vi "Calibration_Main.vi"() -> ()   [LabVIEW 2017]
uses:
  <vilib>/userdefined/High Color/IMAQdx.ctl
  <vilib>/vision/Calibration.llb/Error Statistics.ctl
  Integration/Kicker-XY loop integration/Flow Control Enum.ctl
  <vilib>/vision/NI_Vision_Development_Module.lvlib
panel:
  in  "Tab Control":T1(tab)
  in  "Rebound Only":bool
  out "Kick Success":bool
  out "TrajectorySuccess":bool
  in  "Kick":bool
  in  "stop":bool
  out "error out":errorcluster
  out "ImageOut":T2(plugin-control)
  in  "Session In":T3
  out "X Speed PID":cluster{"Speed SP":dbl, "Speed PV":dbl}(graph)
  out "Y Speed PID":cluster{"Speed SP":dbl, "Speed PV":dbl}(graph)
  out "State":T4(ring)
  out "Kicked":bool
  out "Image":T2(plugin-control)
  out "Datum Check":T5
  in  "EnergyFudgeFactor":dbl
  out "Horizontal Edges":T6(array[cluster]) {"Point2 (Real-World)"."Y" format="%.2f"; "Point2 (Real-World)"."X" format="%.2f"; "Point1 (Real-World)"."Y" format="%.2f"; "Point1 (Real-World)"."X" format="%.2f"; "Point2 (Pixels)"."Y" format="%.2f"; "Point2 (Pixels)"."X" format="%.2f"; "Point1 (Pixels)"."Y" format="%.2f"; "Point1 (Pixels)"."X" format="%.2f"}
  out "Vertical Edges":T6(array[cluster]) {"Point2 (Real-World)"."Y" format="%.2f"; "Point2 (Real-World)"."X" format="%.2f"; "Point1 (Real-World)"."Y" format="%.2f"; "Point1 (Real-World)"."X" format="%.2f"; "Point2 (Pixels)"."Y" format="%.2f"; "Point2 (Pixels)"."X" format="%.2f"; "Point1 (Pixels)"."Y" format="%.2f"; "Point1 (Pixels)"."X" format="%.2f"}
  out "Players":T7(array[cluster]) {"Position"."Y" format="%.2f"; "Position"."X" format="%.2f"}
  out "ChosenAngle":dbl
  out "ChosenPathIdx":i32
  out "ChosenEnergy":dbl
  out "Kicker XY":cluster{dbl, dbl}
  out "Puck":T7(array[cluster]) {"Position"."Y" format="%.2f"; "Position"."X" format="%.2f"}
  out "Image Out":T2(plugin-control)
  out "X 2":sgl
  out "Y 2":sgl
  out "error out 2":errorcluster
  out "Y distance Out":dbl
  out "All Edges Found":bool
  out "X distance":dbl
  out "Histogram Graph":cluster{dbl[], dbl[]}(graph)
  in  "Brightness Input":i64(slide) scale=0.0..255.0
  in  "Contrast Input":dbl(slide) scale=0.0..1.0
  in  "Threshold Input":sgl(slide) scale=0.0..255.0
  in  "Stop":bool
  out "Camera Setup Error":errorcluster
  out "Threshold Image":T2(plugin-control)
  out "Before Image":T2(plugin-control)
  out "Histogram Statistics":T8
  out "Quality Check Variables":T9
  in  "Reference":bool
  in  "stop 2":bool
  out "Image 2":T2(plugin-control)
  in  "Calibrate":bool
  in  "Grid Descriptor":cluster{"X Step":sgl, "Y Step":sgl, "Unit":T10}={"X Step"=5.0, "Y Step"=5.0, "Unit"=enum."Millimeter"}
  in  "File Path":path
  out "Calibration Error":errorcluster
  out "Corrected Image":T2(plugin-control)
  out "Y":sgl
  out "X":sgl
  out "Error Statistics":T11
  # "0.6"
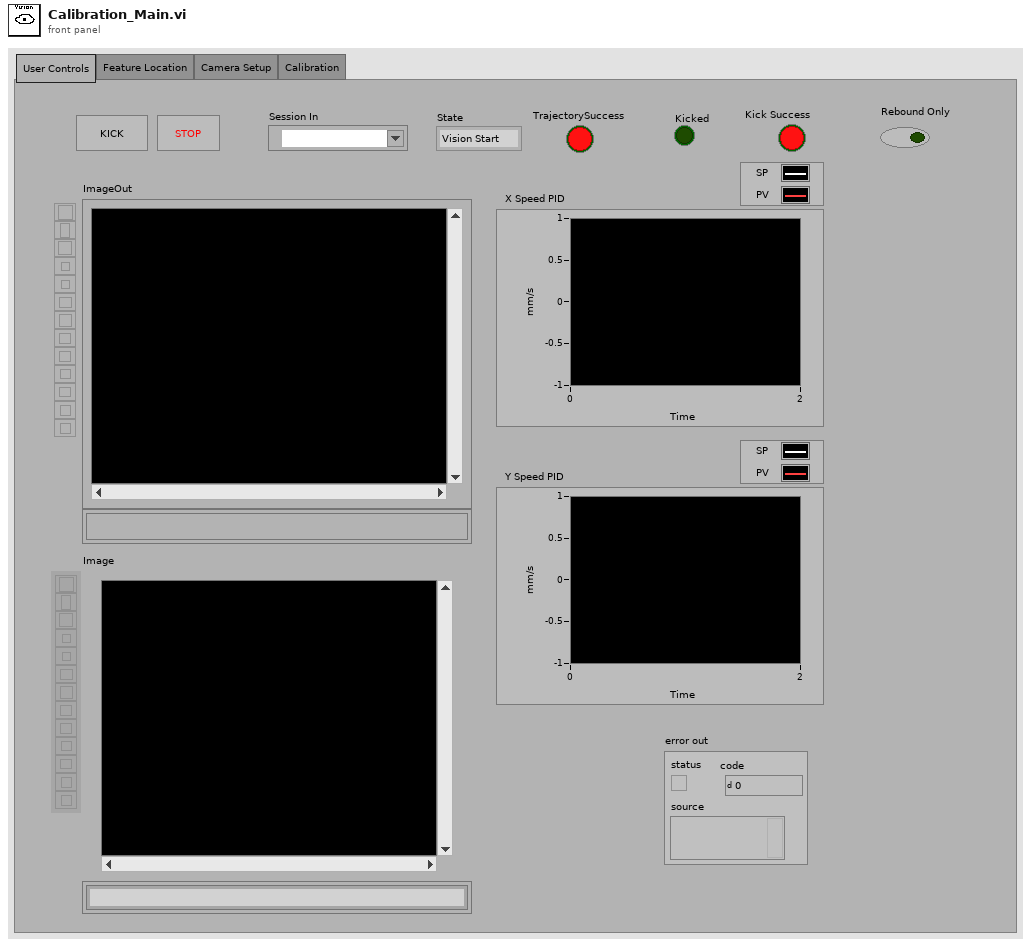
[diagram p1: front panel]
types:
  T1 = enum32{"User Controls", "Feature Location", "Camera Setup", "Calibration"}
  T2 = typedef "IMAQ Image.ctl" = refnum<image>
  T3 = typedef "IMAQdx.ctl" = refnum<k21>
  T4 = enum16{"Vision Start", "Vision End", "Plotting", "Wait"}
  T5 = cluster{"X Coord Correct":bool, "Y Coord Correct":bool}
  T6 = cluster{"Point1 (Pixels)":cluster{"X":sgl, "Y":sgl}, "Point2 (Pixels)":cluster{"X":sgl, "Y":sgl}, "Point1 (Real-World)":cluster{"X":sgl, "Y":sgl}, "Point2 (Real-World)":cluster{"X":sgl, "Y":sgl}, "Angle (Pixel)":dbl, "Angle (Real-World)":dbl, "Score":dbl, "Straightness":dbl, "Average SNR (db)":dbl, "Calibration Valid":bool}[]
  T7 = cluster{"Position":cluster{"X":sgl, "Y":sgl}, "Radius":dbl, "Score":dbl}[]
  T8 = cluster{"Mean Value":sgl, "Standard  Variation":sgl, "Range":sgl}
  T9 = cluster{"Mean +":dbl, "Mean -":dbl, "Within Range":bool}
  T10 = typedef "Image Unit" = enum32{"Undefined", "Angström", "Micrometer", "Millimeter", "Centimeter", "Meter", "Kilometer", "Microinch", "Inch", "Feet", "Nautical miles", "Standard miles", "Steps"}
  T11 = typedef "Error Statistics.ctl" = cluster{"Mean Error":dbl, "Maximum Error":dbl, "Standard Deviation":dbl, "% Distortion":dbl}
  T12 = cluster{"Brightness":i64, "Contrast":dbl, "Threshold":sgl}
  T13 = cluster{"XCoordCorrect":bool, "YCoordCorrect":bool}
  T14 = typedef "IMAQ Coordinate System" = cluster{"Reference System":cluster{"Origin":cluster{"X":sgl, "Y":sgl}, "Angle (deg)":sgl, "Axis Reference":u32}, "Measurement System":cluster{"Origin":cluster{"X":sgl, "Y":sgl}, "Angle (deg)":sgl, "Axis Reference":u32}}
  T15 = cluster{"Circles[0]":cluster{"Position":cluster{"X":sgl, "Y":sgl}, "Radius":dbl, "Score":dbl}, "Circles[1]":cluster{"Position":cluster{"X":sgl, "Y":sgl}, "Radius":dbl, "Score":dbl}, "Circles[2]":cluster{"Position":cluster{"X":sgl, "Y":sgl}, "Radius":dbl, "Score":dbl}, "Circles[3]":cluster{"Position":cluster{"X":sgl, "Y":sgl}, "Radius":dbl, "Score":dbl}, "Circles[4]":cluster{"Position":cluster{"X":sgl, "Y":sgl}, "Radius":dbl, "Score":dbl}, "Circles[5]":cluster{"Position":cluster{"X":sgl, "Y":sgl}, "Radius":dbl, "Score":dbl}, "Circles[6]":cluster{"Position":cluster{"X":sgl, "Y":sgl}, "Radius":dbl, "Score":dbl}, "Circles[7]":cluster{"Position":cluster{"X":sgl, "Y":sgl}, "Radius":dbl, "Score":dbl}, "Circles[8]":cluster{"Position":cluster{"X":sgl, "Y":sgl}, "Radius":dbl, "Score":dbl}}
  T16 = cluster{"X Coord":dbl, "Y Coord":dbl, "Energy":dbl, "Theta Angle":dbl}
  T17 = cluster{"Ptwx":dbl[], "Ptwy":dbl[], "Ptfx":dbl[], "Ptfy":dbl[], "DorR":i32[]}
  T18 = cluster{"X Axis":cluster{"Displacement":dbl, "Speed SP":dbl, "Speed PV":dbl, "Acceleration":dbl}, "Y Axis":cluster{"Displacement":dbl, "Speed SP":dbl, "Speed PV":dbl, "Acceleration":dbl}, "XY Complete?":bool}
  T19 = cluster{"Displacement":dbl, "Speed SP":dbl, "Speed PV":dbl, "Acceleration":dbl}
  T20 = typedef "Flow Control Enum.ctl" = enum16{"Update I/O", "Kicker", "XY Drive", "Theta Axis", "Solenoid", "Go Home"}
  T21 = cluster{"Kicked?":bool, "Stop?":bool, "State":T20, "At Home":bool}
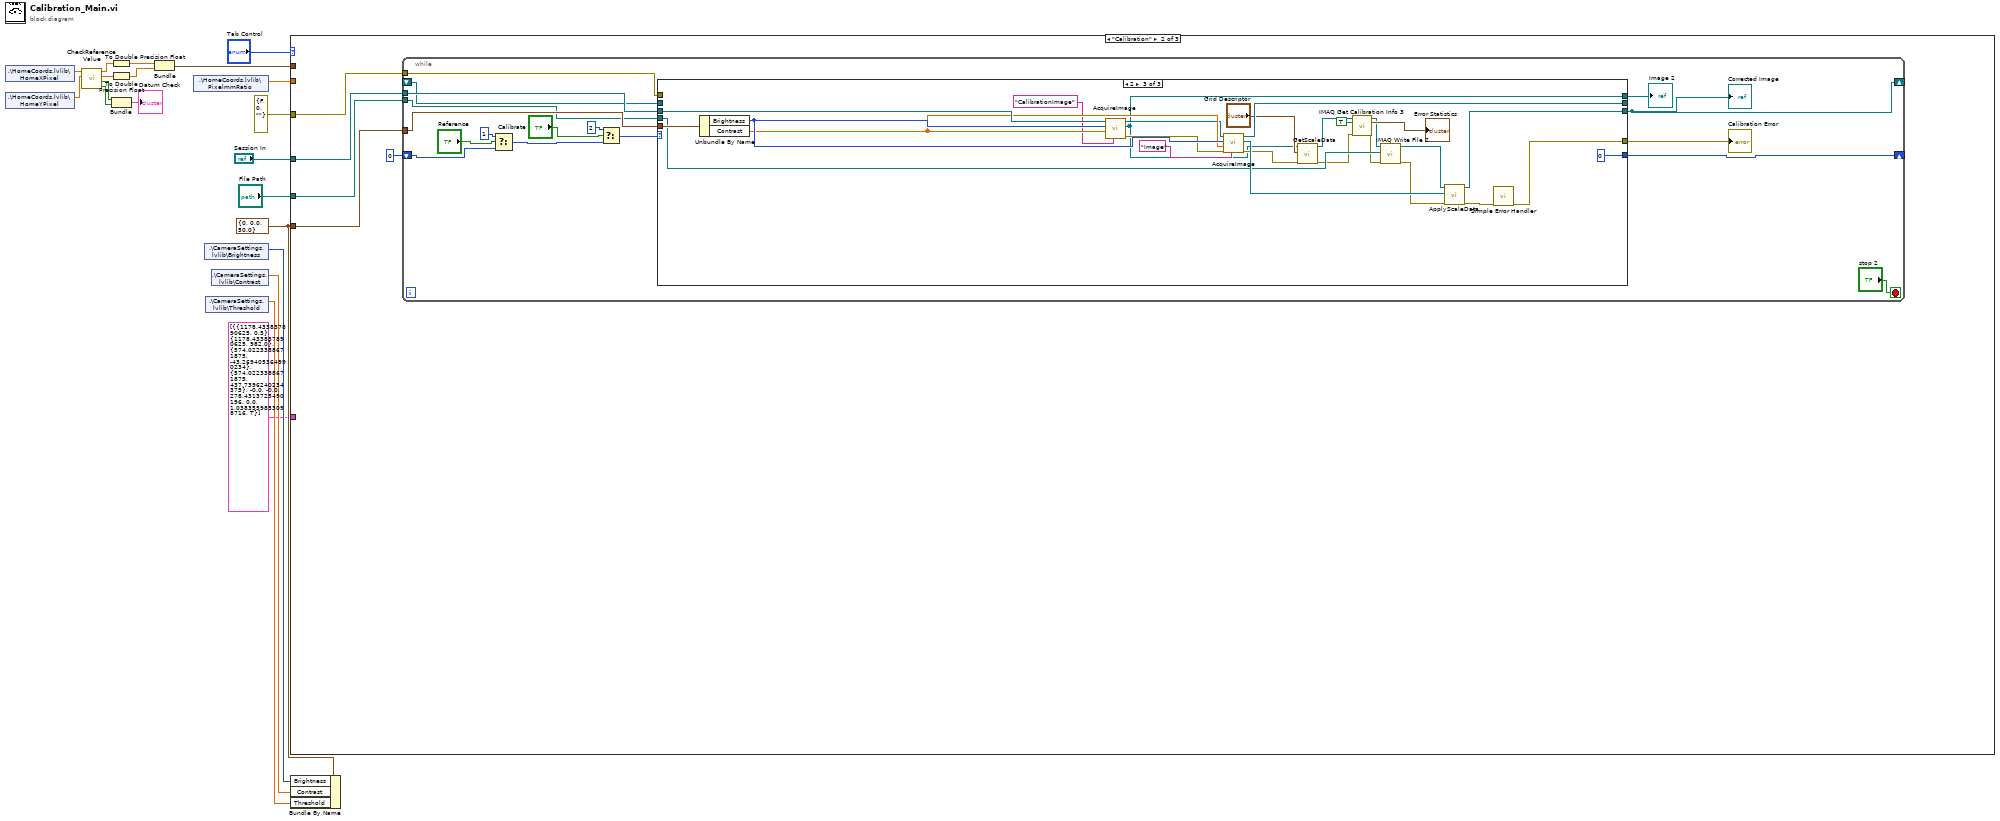
[diagram p0: block diagram]
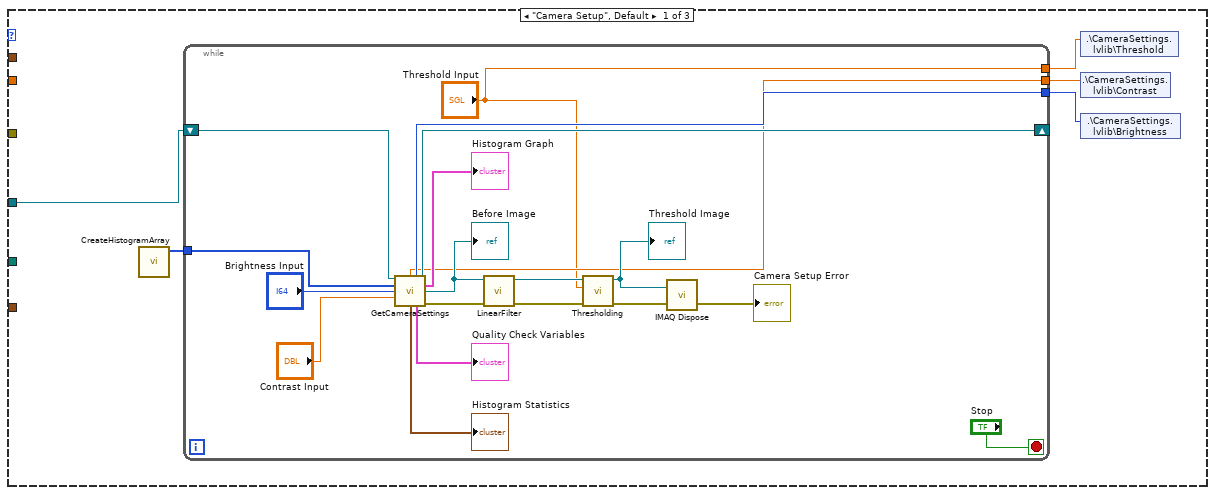
[diagram p2: hidden frame]
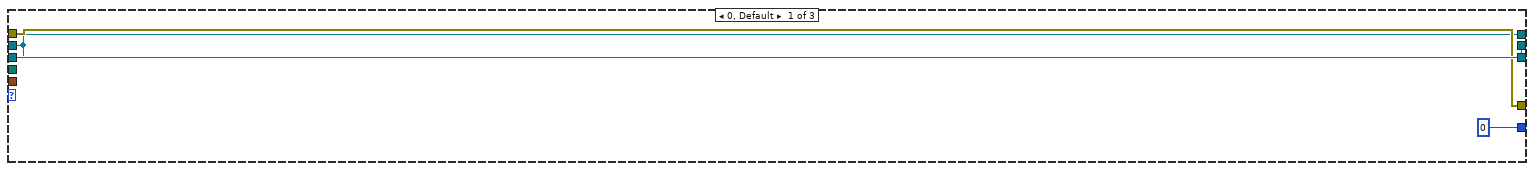
[diagram p3: hidden frame]
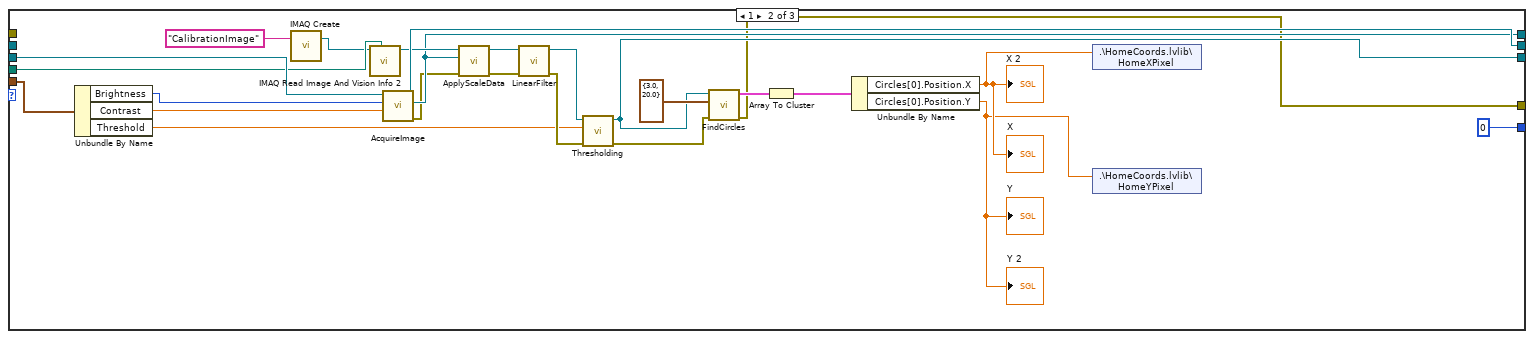
[diagram p4: hidden frame]
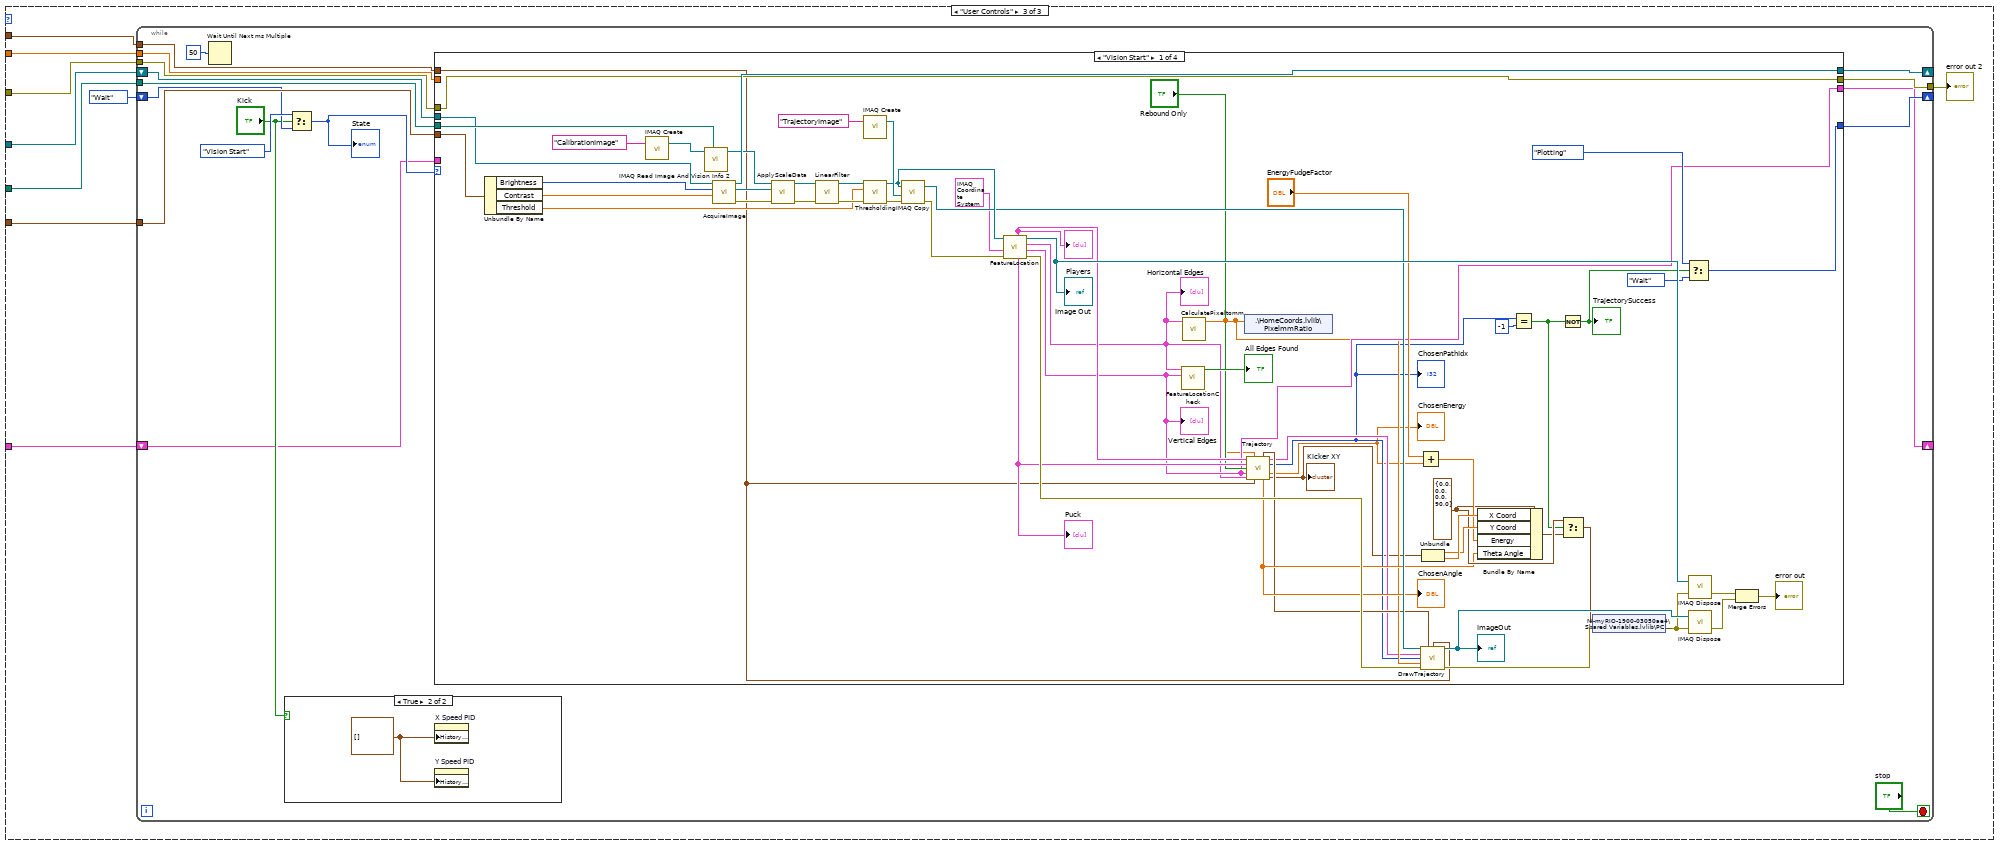
[diagram p5: hidden frame]
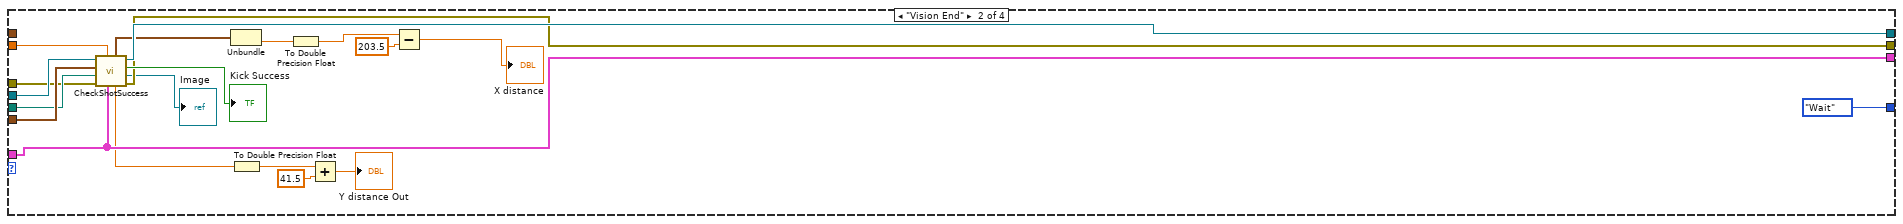
[diagram p7: hidden frame]
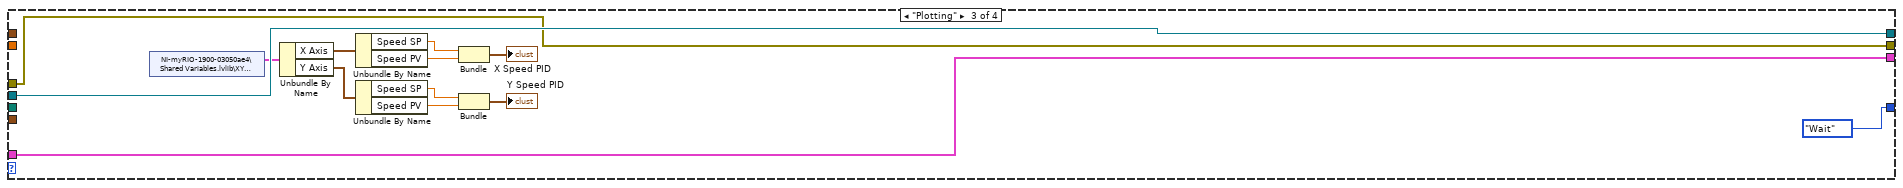
[diagram p8: hidden frame]
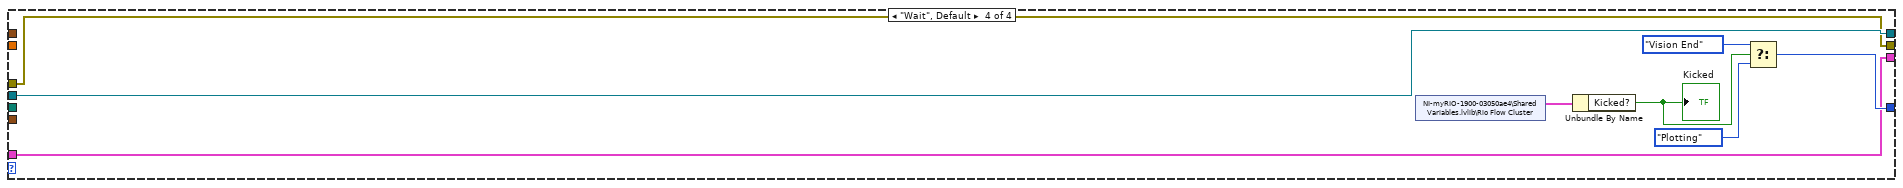
[diagram p9: hidden frame]
diagram:
  w15 = T12 {"Brightness"=0, "Contrast"=0.0, "Threshold"=50.0} ("CameraSettings")
  n1 = shared-variable ".\\HomeCoords.lvlib\\HomeXPixel"() -> (w10:sgl)  [unwired: 1 in, 1 out]
  n2 = shared-variable ".\\HomeCoords.lvlib\\HomeYPixel"() -> (w8:sgl)  [unwired: 1 in, 1 out]
  n3 = call "CheckReferenceValue.vi"("YCoordIn"=w8, "XCoordIn"=w10) -> ("YCoordCorrect"=w2:bool, "XCoordCorrect"=w3:bool, "YCoordOut"=w7:sgl, "XCoordOut"=w9:sgl)  [unwired: 6 in]
  n4 = To Double Precision Float(number=w9) -> (double precision float=w12:dbl)
  n5 = To Double Precision Float(number=w7) -> (double precision float=w11:dbl)
  n6 = Bundle("XCoordCorrect"=w3, "YCoordCorrect"=w2) -> (→"Datum Check":T13)  [unwired: 1 in]
  n7 = Bundle(w12, w11) -> (w17:cluster{dbl, dbl})  [unwired: 1 in]
  n8 = shared-variable ".\\HomeCoords.lvlib\\PixelmmRatio"() -> (w5:dbl)  [unwired: 1 in, 1 out]
  n9 = shared-variable ".\\CameraSettings.lvlib\\Brightness"() -> (w16:i64)  [unwired: 1 in, 1 out]
  n10 = shared-variable ".\\CameraSettings.lvlib\\Threshold"() -> (w13:sgl)  [unwired: 1 in, 1 out]
  n11 = shared-variable ".\\CameraSettings.lvlib\\Contrast"() -> (w14:dbl)  [unwired: 1 in, 1 out]
  n12 = case shown="\"Calibration\"" "Tab Control" {
    tunnel: "Session In" -> [w24 w49 w130]
    tunnel: w15 -> [_ w48 w128]
    tunnel: "File Path" -> [_ w47 w129]
    tunnel: errorcluster {"status"=FALSE, "code"=0, "source"=""} ("error out") -> [_ w45 w126]
    tunnel: w17 -> [_ _ w127]
    tunnel: w5 -> [_ _ w123]
    tunnel: T6 [{"Point1 (Pixels)"={"X"=1178.4338, "Y"=0.5}, "Point2 (Pixels)"={"X"=1178.4338, "Y"=982.0}, "Point1 (Real-World)"={"X"=574.02234, "Y"=-43.269405}, "Point2 (Real-World)"={"X"=574.02234, "Y"=437.73962}, "Angle (Pixel)"=-0.0, "Angle (Real-World)"=-0.0, "Score"=278.4313725490196, "Straightness"=0.0, "Average SNR (db)"=1.0383559853098716, "Calibration Valid"=TRUE}] ("Vertical Edges 2") -> [_ _ w122]
    frame "Camera Setup", Default {
      n13 = call "CreateHistogramArray.vi"() -> ("Array"=w25:i32[])  [unwired: 11 in]
      n14 = while {
        shift-right: [w34] -> _
        shift-left: w24 -> [w42]
        tunnel: w25 -> [w41]
        tunnel: [w29] -> w22
        tunnel: ["Threshold Input"] -> w21
        tunnel: [w30] -> w23
        stop <- "Stop" stop-if-true
        n15 = call "GetCameraSettings.vi"("Session In"=w42, "Array"=w41, "Brightness"="Brightness Input", "Contrast"="Contrast Input") -> ("Contrast"=w29:dbl, "Brightness"=w30:i64, "Session Out"=w34:T3, "Histogram Graph"=→"Histogram Graph":cluster{dbl[], dbl[]}, "Image"=w33:T2, "Histogram Statistics"=→"Histogram Statistics":T8, "Quality Check Variables"=→"Quality Check Variables":T9, "error out"=w32:errorcluster)  [unwired: 4 in]
        "Before Image" <- w33
        n16 = call "LinearFilter.vi"("error in (no error)"=w32, "Image Src"=w33) -> ("error out"=w37:errorcluster, "Image"=w38:T2)  [unwired: 8 in]
        n17 = call "Thresholding.vi"("error in (no error)"=w37, "Threshold Value"="Threshold Input", "Image Src"=w38) -> ("error out"=w36:errorcluster, "Image"=w35:T2)  [unwired: 7 in]
        "Threshold Image" <- w35
        n18 = call "IMAQ Dispose"("Image"=w35, "error in (no error)"=w36) -> ("error out"=→"Camera Setup Error":errorcluster)  [unwired: 4 in]
      }
      n19 = shared-variable ".\\CameraSettings.lvlib\\Threshold"(w21) -> ()  [unwired: 1 in, 1 out]
      n20 = shared-variable ".\\CameraSettings.lvlib\\Contrast"(w22) -> ()  [unwired: 1 in, 1 out]
      n21 = shared-variable ".\\CameraSettings.lvlib\\Brightness"(w23) -> ()  [unwired: 1 in, 1 out]
    }
    frame "Calibration" {
      n22 = while {
        tunnel: w49 -> [w66]
        tunnel: w48 -> [w65]
        tunnel: w47 -> [w63]
        shift-right: [w62] -> _
        shift-left: 0 -> [w56]
        shift-right: [w50] -> _
        shift-left: _ -> [w53]
        tunnel: w45 -> [w54]
        stop <- "stop 2" stop-if-true
        n23 = Select(t=1, s="Reference", f=w56) -> (s? t:f=w59:i32)
        n24 = Select(t=2, s="Calibrate", f=w59) -> (s? t:f=w55:i32)
        n25 = case shown="2" w55 {
          tunnel: w66 -> [w70 w93 w121]
          tunnel: w65 -> [_ w91 w120]
          tunnel: [w70 w92 w113] -> _
          tunnel: w63 -> [_ w89 w105]
          tunnel: [w68 w73 w115] -> w52
          tunnel: [w67 w74 w106] -> w50
          tunnel: [0 0 0] -> w62
          tunnel: w54 -> [w68 _ _]
          tunnel: w53 -> [w67 _ _]
          tunnel: [w67 w85 w104] -> w51
          frame 0, Default {
          }
          frame 1 {
            n26 = Unbundle By Name(w91) -> ("Brightness"=w95:i64, "Contrast"=w94:dbl, "Threshold"=w79:sgl)
            n27 = call "IMAQ Create"("Image Name"="CalibrationImage") -> ("New Image"=w87:T2)  [unwired: 4 in, 1 out]
            n28 = call "IMAQ Read Image And Vision Info 2"("File Path"=w89, "Image"=w87) -> ("Image Out"=w86:T2)  [unwired: 7 in, 2 out]
            n29 = call "AcquireImage.vi"("Contrast"=w94, "Brightness"=w95, "Session In"=w93) -> ("error out"=w82:errorcluster, "Image"=w85:T2, "Session Out"=w92:T3)  [unwired: 5 in]
            n30 = call "ApplyScaleData.vi"("error in (no error)"=w82, "ImageIn"=w85, "CalibImage"=w86) -> ("error out"=w81:errorcluster, "Corrected Image"=w84:T2)  [unwired: 7 in]
            n31 = call "LinearFilter.vi"("error in (no error)"=w81, "Image Src"=w84) -> ("error out"=w80:errorcluster, "Image"=w83:T2)  [unwired: 8 in]
            n32 = call "Thresholding.vi"("error in (no error)"=w80, "Threshold Value"=w79, "Image Src"=w83) -> ("error out"=w77:errorcluster, "Image"=w74:T2)  [unwired: 7 in]
            n33 = call "FindCircles.vi"("error in (no error)"=w77, "Circle Descriptor"=cluster{"Min Radius":dbl, "Max Radius":dbl} {"Min Radius"=3.0, "Max Radius"=20.0}, "Image"=w74) -> ("error out"=w73:errorcluster, "Circles"=w76:T7)  [unwired: 6 in, 1 out]
            n34 = Array To Cluster(array=w76) -> (cluster=w75:T15)
            n35 = Unbundle By Name(w75) -> ("Circles[0].Position.X"=w72:sgl, "Circles[0].Position.Y"=w71:sgl)
            "X 2" <- w72
            "Y 2" <- w71
            "Y" <- w71
            "X" <- w72
            n36 = shared-variable ".\\HomeCoords.lvlib\\HomeXPixel"(w72) -> ()  [unwired: 1 in, 1 out]
            n37 = shared-variable ".\\HomeCoords.lvlib\\HomeYPixel"(w71) -> ()  [unwired: 1 in, 1 out]
          }
          frame 2 {
            n38 = Unbundle By Name(w120) -> ("Brightness"=w118:i64, "Contrast"=w117:dbl)
            n39 = call "AcquireImage.vi"("Image Name"="CalibrationImage", "Contrast"=w117, "Brightness"=w118, "Session In"=w121) -> ("error out"=w116:errorcluster, "Image"=w104:T2, "Session Out"=w114:T3)  [unwired: 4 in]
            n40 = call "AcquireImage.vi"("Image Name"="Image", "error in"=w116, "Contrast"=w117, "Brightness"=w118, "Session In"=w114) -> ("error out"=w108:errorcluster, "Image"=w109:T2, "Session Out"=w113:T3)  [unwired: 3 in]
            n41 = call "GetScaleData.vi"("error in (no error)"=w108, "Grid Descriptor"="Grid Descriptor", "Image Src"=w104) -> ("error out"=w99:errorcluster, "Image"=w102:T2)  [unwired: 7 in]
            n42 = call "IMAQ Get Calibration Info 3"("Calibration Template Image"=w102, "Return Error Information (False)"=TRUE, "error in (no error)"=w99) -> ("Calibration Template Image (duplicate)"=w100:T2, "Error Statistics"=→"Error Statistics":T11, "error out"=w98:errorcluster)  [unwired: 4 in, 6 out]
            n43 = call-poly "IMAQ Write File 2"("error in (no error)"=w98, "File Path"=w105, "Image"=w100) -> ("error out"=w97:errorcluster, "Image Out (duplicate)"=w101:T2)  [unwired: 7 in]
            n44 = call "ApplyScaleData.vi"("error in (no error)"=w97, "ImageIn"=w109, "CalibImage"=w101) -> ("error out"=w107:errorcluster, "Corrected Image"=w106:T2)  [unwired: 7 in]
            n45 = call <vilib>:"Simple Error Handler.vi"("error in (no error)"=w107) -> ("error out"=w115:errorcluster)  [unwired: 4 in, 4 out]
          }
        }
        "Calibration Error" <- w52
        "Image 2" <- w51
        "Corrected Image" <- w50
      }
    }
    frame "User Controls" {
      n46 = while {
        shift-right: [w146] -> _
        shift-left: w130 -> [w147]
        tunnel: w129 -> [w144]
        tunnel: w128 -> [w143]
        tunnel: w127 -> [w142]
        shift-right: [w139] -> _
        shift-left: T4."Wait" -> [w138]
        tunnel: w126 -> [w135]
        tunnel: [w134] -> w125
        tunnel: w123 -> [w133]
        shift-right: [w131] -> _
        shift-left: w122 -> [w132]
        stop <- "stop" stop-if-true
        n47 = Wait Until Next ms Multiple(millisecond multiple=u32 50) -> ()  [unwired: 1 out]
        n48 = case shown="True" "Kick" {
          frame False {
          }
          frame True {
            w148 = cluster{"Speed SP":dbl, "Speed PV":dbl}[] [] ("History Data")
            n49 = property on="X Speed PID" class="WFChart (strict)"("History Data"=w148) -> ()  [unwired: 2 in, 2 out]
            n50 = property on="Y Speed PID" class="WFChart (strict)"("History Data"=w148) -> ()  [unwired: 2 in, 2 out]
          }
        }
        n51 = Select(t=T4."Vision Start", s="Kick", f=w138) -> (s? t:f=w140:T4)
        "State" <- w140
        n52 = case shown="\"Vision Start\"" w140 {
          tunnel: w147 -> [w195 w226 w240 w248]
          tunnel: [w204 w225 w240 w248] -> w146
          tunnel: w144 -> [w207 w221 _ _]
          tunnel: w143 -> [w202 w222 _ _]
          tunnel: w142 -> [w156 _ _ _]
          tunnel: [w164 T4."Wait" T4."Wait" w244] -> w139
          tunnel: w135 -> [w163 w220 w230 w247]
          tunnel: [w163 w219 w230 w247] -> w134
          tunnel: w133 -> [_ w223 _ _]
          tunnel: w132 -> [_ w218 w228 w241]
          tunnel: [w158 w218 w228 w241] -> w131
          frame "Vision Start" {
            w171 = T16 {"X Coord"=0.0, "Y Coord"=0.0, "Energy"=0.0, "Theta Angle"=90.0} ("PC To Rio")
            n53 = Unbundle By Name(w202) -> ("Brightness"=w194:i64, "Contrast"=w193:dbl, "Threshold"=w198:sgl)
            n54 = call "IMAQ Create"("Image Name"="CalibrationImage") -> ("New Image"=w205:T2)  [unwired: 4 in, 1 out]
            n55 = call "IMAQ Read Image And Vision Info 2"("File Path"=w207, "Image"=w205) -> ("Image Out"=w203:T2)  [unwired: 7 in, 2 out]
            n56 = call "AcquireImage.vi"("Contrast"=w193, "Brightness"=w194, "Session In"=w195) -> ("error out"=w196:errorcluster, "Image"=w192:T2, "Session Out"=w204:T3)  [unwired: 5 in]
            n57 = call "ApplyScaleData.vi"("error in (no error)"=w196, "ImageIn"=w192, "CalibImage"=w203) -> ("error out"=w200:errorcluster, "Corrected Image"=w197:T2)  [unwired: 7 in]
            n58 = call "LinearFilter.vi"("error in (no error)"=w200, "Image Src"=w197) -> ("error out"=w199:errorcluster, "Image"=w201:T2)  [unwired: 8 in]
            n59 = call "IMAQ Create"("Image Name"="TrajectoryImage") -> ("New Image"=w190:T2)  [unwired: 4 in, 1 out]
            n60 = call "Thresholding.vi"("error in (no error)"=w199, "Threshold Value"=w198, "Image Src"=w201) -> ("error out"=w188:errorcluster, "Image"=w185:T2)  [unwired: 7 in]
            n61 = call "IMAQ Copy"("error in (no error)"=w188, "Image Dst"=w190, "Image Src"=w185) -> ("error out"=w187:errorcluster, "Image Dst Out"=w183:T2)  [unwired: 3 in]
            n62 = call "FeatureLocation.vi"("error in (no error)"=w187, "Coordinate System"=T14 {"Reference System"={"Origin"={"X"=0.0, "Y"=0.0}, "Angle (deg)"=0.0, "Axis Reference"=0}, "Measurement System"={"Origin"={"X"=0.0, "Y"=0.0}, "Angle (deg)"=0.0, "Axis Reference"=0}}, "Image"=w185) -> ("error out"=w186:errorcluster, "Vertical Edges"=w158:T6, "Horizontal Edges"=w157:T6, "Image 2"=w184:T2, "Puck"=w160:T7, "Players"=w161:T7)  [unwired: 3 in]
            "Image Out" <- w184
            "Horizontal Edges" <- w157
            "Vertical Edges" <- w158
            "Players" <- w161
            "Puck" <- w160
            n63 = call "FeatureLocationCheck.vi"("Vertical Edges"=w158, "Horizontal Edges"=w157) -> ("All Edges Found"=→"All Edges Found":bool)  [unwired: 9 in]
            n64 = call "CalculatePixeltomm.vi"("Horizontal Edges"=w157) -> ("Pixel/mm"=w154:dbl)  [unwired: 10 in]
            n65 = shared-variable ".\\HomeCoords.lvlib\\PixelmmRatio"(w154) -> ()  [unwired: 1 in, 1 out]
            n66 = call "Trajectory.vi"("Players"=w161, "PixelmmRatio"=w154, "Puck"=w160, "Rebound Only"="Rebound Only", "Vertical Edges"=w158, "Horizontal Edges"=w157, "HomeXY(pixels)"=w156) -> ("PuckCentre"=w153:cluster{"PuckX":sgl, "PuckY":sgl}, "TrajectoryArray"=w152:T17, "ChosenPathIdx"=w151:i32, "ChosenEnergy"=w150:dbl, "Angle"=w155:dbl, "Kicker XY"=w149:cluster{dbl, dbl})  [unwired: 3 in]
            "ChosenPathIdx" <- w151
            "ChosenEnergy" <- w150
            "Kicker XY" <- w149
            "ChosenAngle" <- w155
            n67 = Add(x="EnergyFudgeFactor", y=w150) -> (x+y=w174:dbl)
            n68 = call "DrawTrajectory.vi"("Image"=w183, "PuckCentre"=w153, "HomePoint(pixels)"=w156, "TrajectoryArray"=w152, "ChosenPath"=w151, "Pixel/mm"=w154, "error in (no error)"=w186) -> ("ImageOut"=w189:T2, "error out"=w176:errorcluster)  [unwired: 7 in]
            "ImageOut" <- w189
            n69 = Unbundle(w149) -> (w180:dbl, w181:dbl)
            n70 = Bundle By Name(cluster=w171, "X Coord"=w181, "Y Coord"=w180, "Energy"=w174, "Theta Angle"=w155) -> (w170:T16)
            n71 = Equal?(x=w151, y=-1) -> (x = y?=w168:bool)
            n72 = Not(x=w168) -> (.not. x?=w167:bool)
            "TrajectorySuccess" <- w167
            n73 = Select(t=w171, s=w168, f=w170) -> (s? t:f=w169:T16)
            n74 = shared-variable "NI-myRIO-1900-03050ae4\\Shared Variables.lvlib\\PC To Rio"(w169, error in=w176) -> (error out=w175:errorcluster)
            n75 = Select(t=T4."Plotting", s=w167, f=T4."Wait") -> (s? t:f=w164:T4)
            n76 = call "IMAQ Dispose"("Image"=w184, "error in (no error)"=w175) -> ("error out"=w179:errorcluster)  [unwired: 4 in]
            n77 = call "IMAQ Dispose"("Image"=w189, "error in (no error)"=w175) -> ("error out"=w178:errorcluster)  [unwired: 4 in]
            n78 = Merge Errors(w179, w178) -> (→"error out":errorcluster)
          }
          frame "Vision End" {
            n79 = call "CheckShotSuccess.vi"("Vertical Edges"=w218, "Pixel/mm"=w223, "error in"=w220, "File Path"=w221, "CameraSettings"=w222, "Session In"=w226) -> ("error out"=w219:errorcluster, "Image"=→"Image":T2, "Success?"=→"Kick Success":bool, "Session Out"=w225:T3, "X distance Out"=w215:sgl, "XYPuck"=w212:cluster{sgl, sgl})
            n80 = Unbundle(w212) -> (w208:sgl)  [unwired: 1 out]
            n81 = To Double Precision Float(number=w215) -> (double precision float=w214:dbl)
            n82 = To Double Precision Float(number=w208) -> (double precision float=w209:dbl)
            n83 = Add(x=w214, y=41.5) -> (x+y=→"Y distance Out":dbl)
            n84 = Subtract(x=w209, y=203.5) -> (x-y=→"X distance":dbl)
          }
          frame "Plotting" {
            n85 = shared-variable "NI-myRIO-1900-03050ae4\\Shared Variables.lvlib\\XY Telemetry"() -> (w237:T18)  [unwired: 1 in, 1 out]
            n86 = Unbundle By Name(w237) -> ("X Axis"=w239:T19, "Y Axis"=w238:T19)
            n87 = Unbundle By Name(w239) -> ("Speed SP"=w236:dbl, "Speed PV"=w235:dbl)
            n88 = Unbundle By Name(w238) -> ("Speed SP"=w233:dbl, "Speed PV"=w232:dbl)
            n89 = Bundle("Speed SP"=w236, "Speed PV"=w235) -> (→"X Speed PID":cluster{"Speed SP":dbl, "Speed PV":dbl})  [unwired: 1 in]
            n90 = Bundle("Speed SP"=w233, "Speed PV"=w232) -> (→"Y Speed PID":cluster{"Speed SP":dbl, "Speed PV":dbl})  [unwired: 1 in]
          }
          frame "Wait", Default {
            n91 = shared-variable "NI-myRIO-1900-03050ae4\\Shared Variables.lvlib\\Rio Flow Cluster"() -> (w243:T21)  [unwired: 1 in, 1 out]
            n92 = Unbundle By Name(w243) -> ("Kicked?"=w242:bool)
            "Kicked" <- w242
            n93 = Select(t=T4."Vision End", s=w242, f=T4."Plotting") -> (s? t:f=w244:T4)
          }
        }
      }
      "error out 2" <- w125
    }
  }
  n94 = Bundle By Name(cluster=w15, "Brightness"=w16, "Contrast"=w14, "Threshold"=w13) -> ()  [unwired: 1 out]
